vi "get secure settings.vi"(8 "error in (no error)":errorcluster, 10 "secure_settings":T1, 11 "id":i32) -> (0 "error out":errorcluster, 2 "secure_settings out":T1, 3 "function return":i32)   [LabVIEW 2012, in "libximc.lvlib"]
doc: "result_t XIMC_API get_secure_settings (device_t id, secure_settings_t* secure_settings);"
uses:
  libximc.lvlib
  libximc.dll
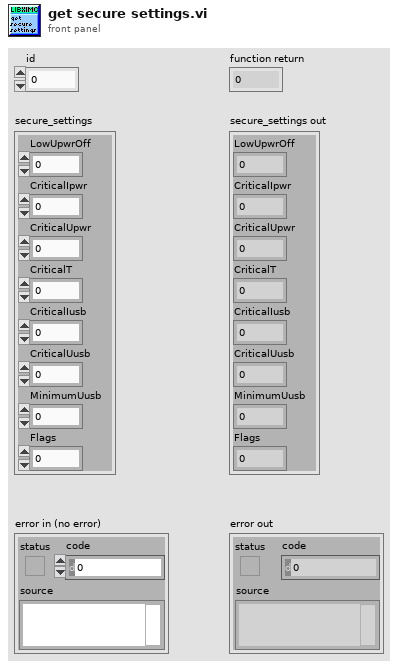
[diagram p1: front panel]
types:
  T1 = cluster{"LowUpwrOff":u32, "CriticalIpwr":u32, "CriticalUpwr":u32, "CriticalT":u32, "CriticalIusb":u32, "CriticalUusb":u32, "MinimumUusb":u32, "Flags":u32}
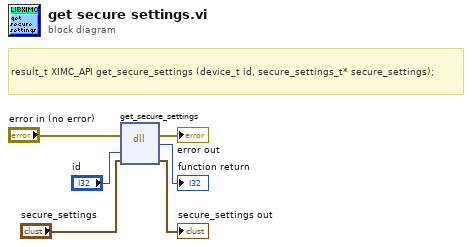
[diagram p0: block diagram]
diagram:
  # "result_t XIMC_API get_secure_settings (device_t id, secure_settings_t* secure_settings);"
  n1 = dll-call lib="C:/Users/Stepan/Downloads/labview_2.9.11_testgen_thread/libximc.*" fn="get_secure_settings"(error in="error in (no error)", "id"="id", "secure_settings"="secure_settings") -> (error out=→"error out":errorcluster, →"function return":i32, "secure_settings"=→"secure_settings out":T1)  [unwired: 3 in, 1 out]
